vi "Teleop.vi"(10 "Match Info":T1={"Autonomous Elapsed Seconds"=0.0, "TeleOp Elapsed Seconds"=0.0, "Disabled Elapsed Seconds"=0.0, "Visited Autonomous"=FALSE, "Visited TeleOp"=FALSE, "Visited Disabled"=FALSE, "Autonomous Settings"={"Autonomous Style"=enum."Independent", "VI Refnum"=refnum}}, 11 "Call Context":T2) -> ()   [LabVIEW 2020]
doc: "This VI is called for each TeleOp packet received from the DS where the robot is not disabled. It is often used to read from the joysticks and update I/O or to update setpoints for timed control loops. It should complete and return within 20 milliseconds or it may miss DS packets."
uses:
  <vilib>/Rock Robotics/WPI/DriverStation/WPI_DriverStationDerivedRobotMode.ctl
  <vilib>/Rock Robotics/WPI/DriverStation/WPI_DriverStationMatch Info.ctl
  <vilib>/Rock Robotics/WPI/Joystick/XBox Buttons Indexer.ctl
  <vilib>/Rock Robotics/WPI/Joystick/XBox Axes Indexer.ctl
  <vilib>/Rock Robotics/Network Tables/NT Read Boolean.vi
  <vilib>/Rock Robotics/Network Tables/NT Read Number.vi
  Auxilary/AuxGlobals.vi
  Climb/ClimbGlobals.vi
  <vilib>/Rock Robotics/Network Tables/NT Write String.vi
  Human/HumanGlobal.vi
  <vilib>/Rock Robotics/Network Tables/NT Write Boolean.vi
  <vilib>/Rock Robotics/WPI/Joystick/WPI_JoystickArcadeMapping.vi
  <vilib>/Rock Robotics/WPI/ThirdParty/JAS_Junk/TrajLib/Trajectory_Library.lvlib
panel:
  out "Sample Slider 0":dbl(slide) scale=0.0..5.0
  out "Sample Boolean 1":bool
  out "Sample Boolean 0":bool
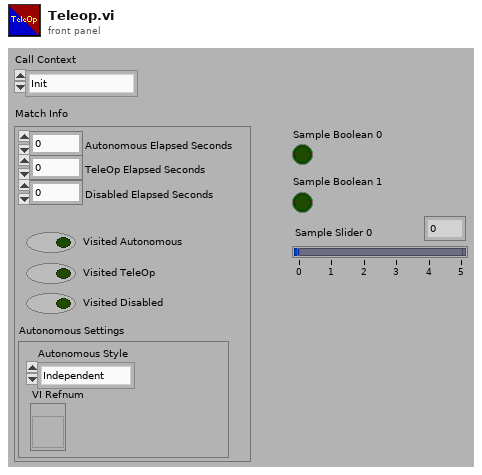
[diagram p1: front panel]
types:
  T1 = typedef "WPI_DriverStationMatch Info.ctl" = cluster{"Autonomous Elapsed Seconds":dbl, "TeleOp Elapsed Seconds":dbl, "Disabled Elapsed Seconds":dbl, "Visited Autonomous":bool, "Visited TeleOp":bool, "Visited Disabled":bool, "Autonomous Settings":cluster{"Autonomous Style":enum16{"Iterative", "Independent"}, "VI Refnum":refnum<vi>}}
  T2 = typedef "WPI_DriverStationDerivedRobotMode.ctl" = enum16{"Init", "Execute", "Stop"}
  T3 = typedef "XBox Buttons Indexer.ctl" = enum16{"A", "B", "X", "Y", "Left Bumper", "Right Bumper", "Back", "Start", "Left Joystick", "Right Joystick"}
  T4 = typedef "XBox Axes Indexer.ctl" = enum16{"Left X", "Left Y", "Left Trigger", "Right Trigger", "Right X", "Right Y"}
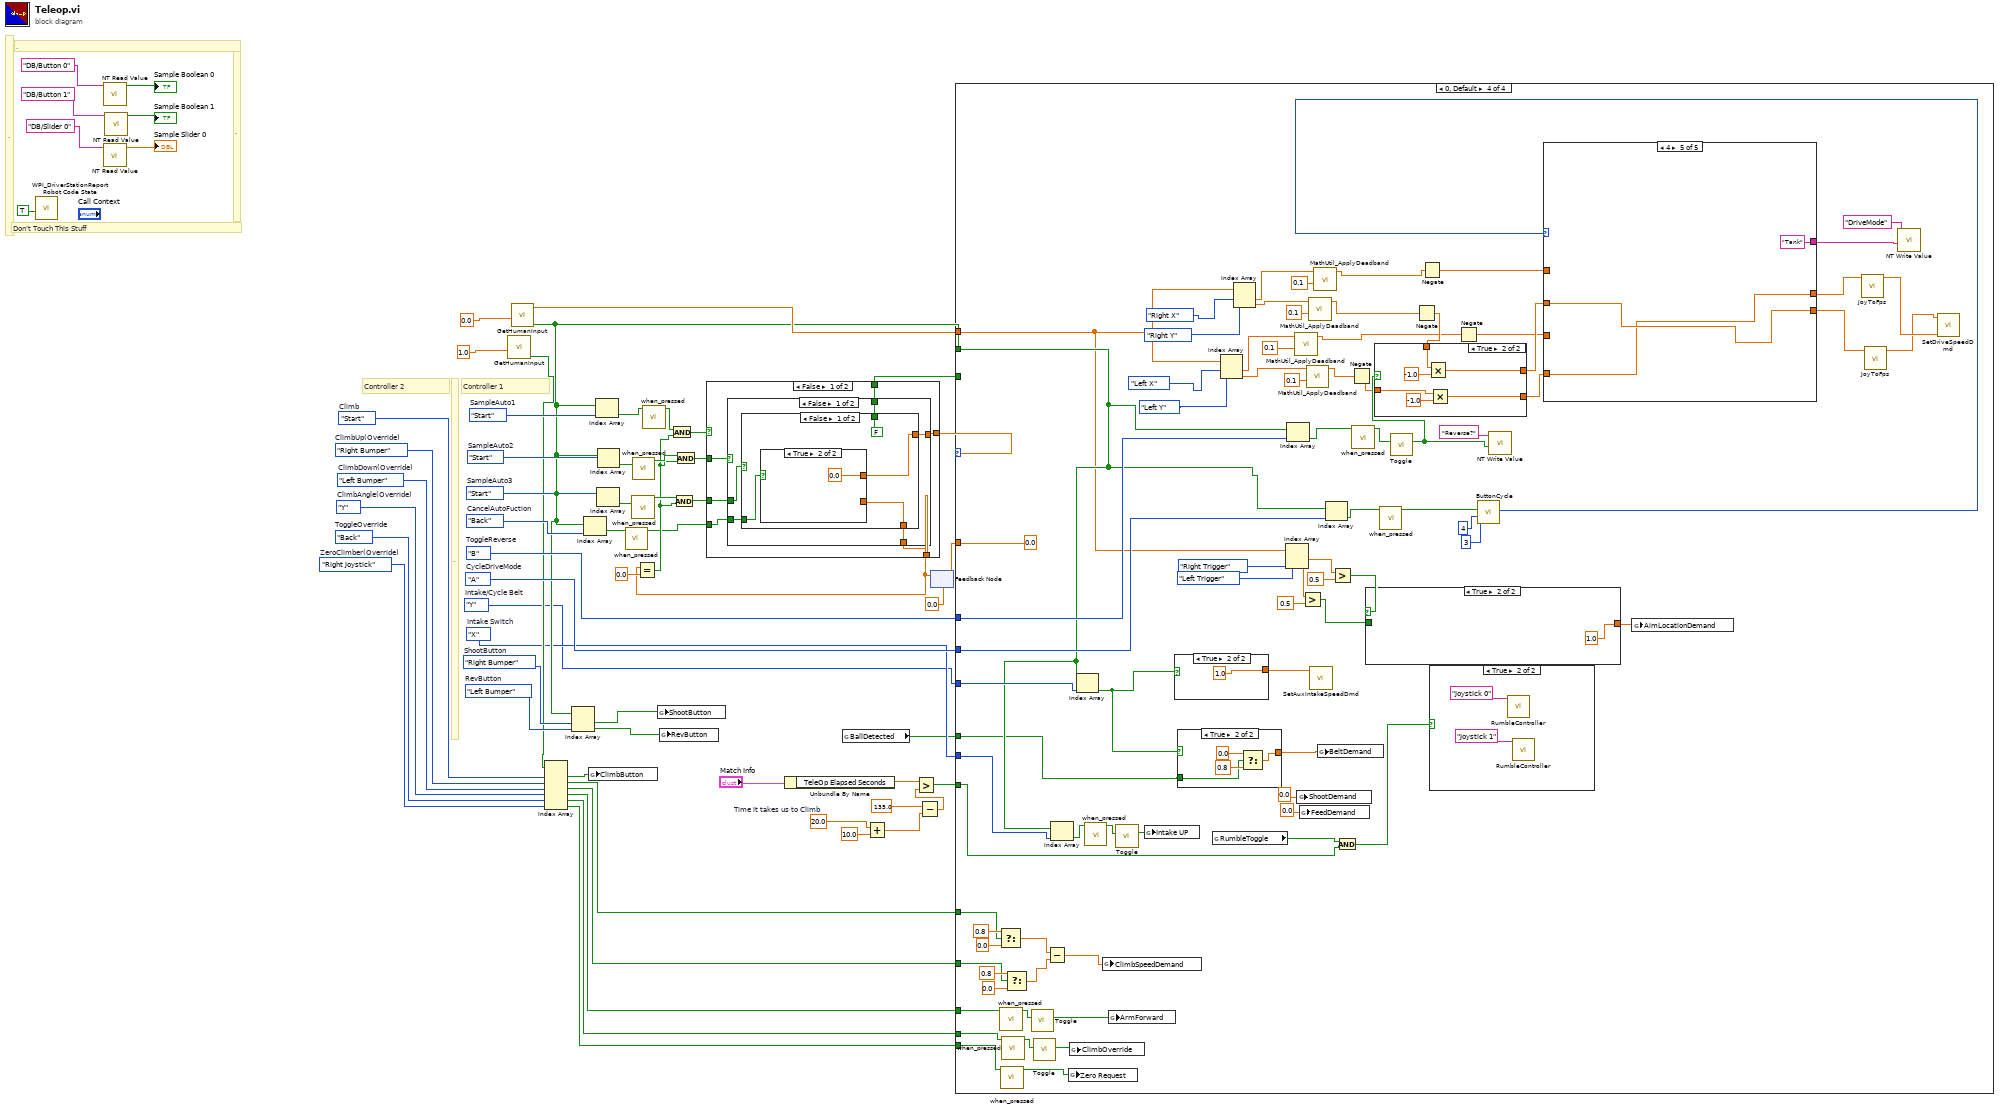
[diagram p0: block diagram]
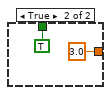
[diagram p3: hidden frame]
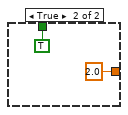
[diagram p4: hidden frame]
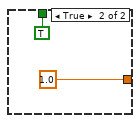
[diagram p5: hidden frame]
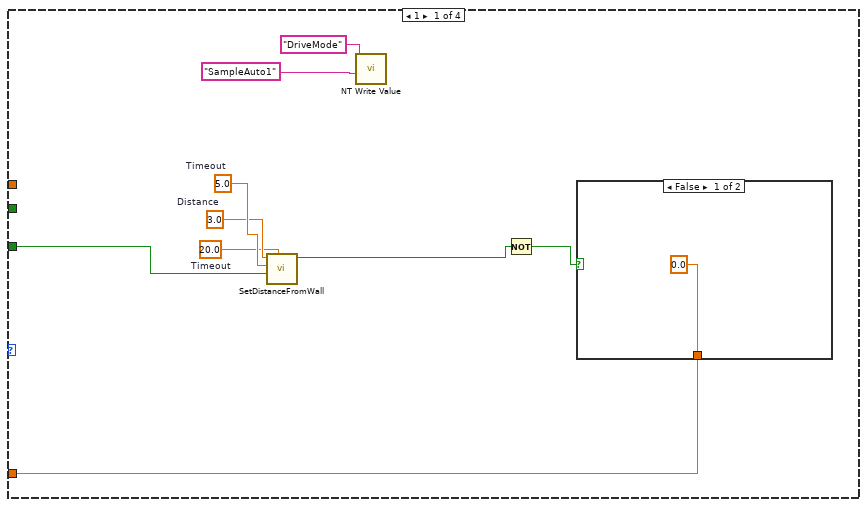
[diagram p6: hidden frame]
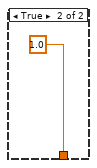
[diagram p7: hidden frame]
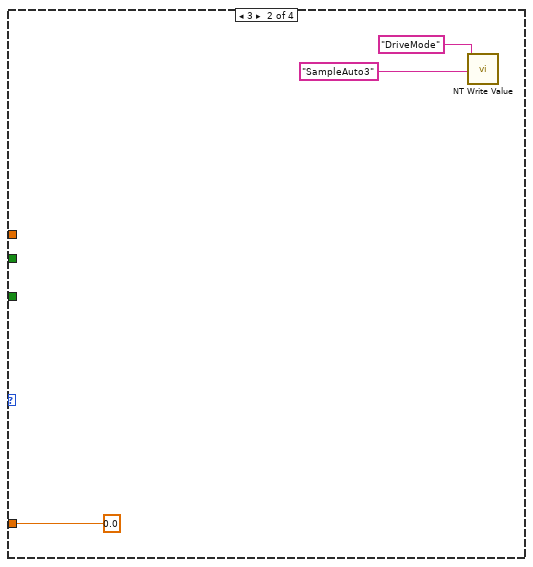
[diagram p8: hidden frame]
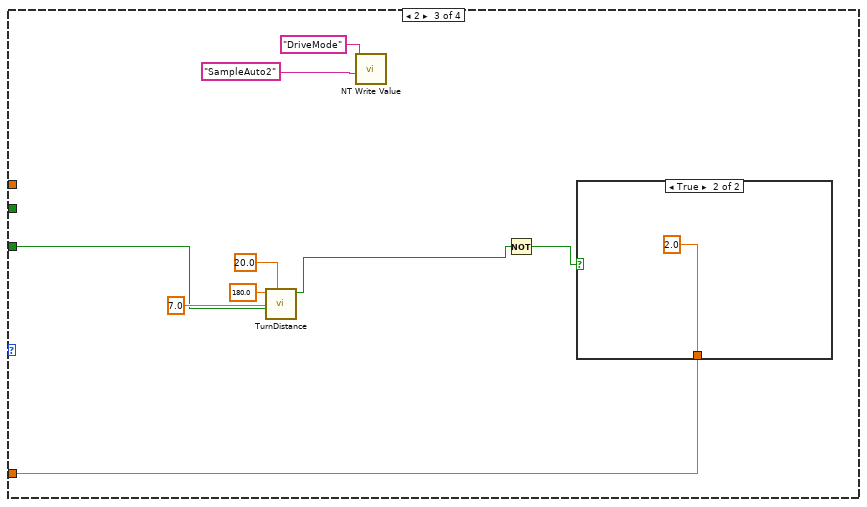
[diagram p9: hidden frame]
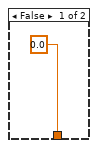
[diagram p10: hidden frame]
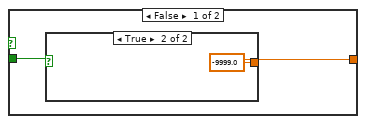
[diagram p11: hidden frame]
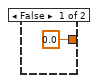
[diagram p12: hidden frame]
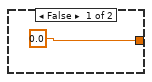
[diagram p13: hidden frame]
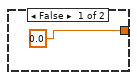
[diagram p14: hidden frame]
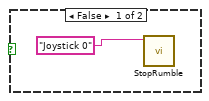
[diagram p15: hidden frame]
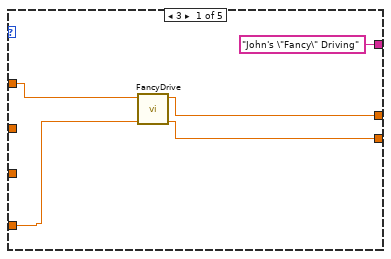
[diagram p17: hidden frame]
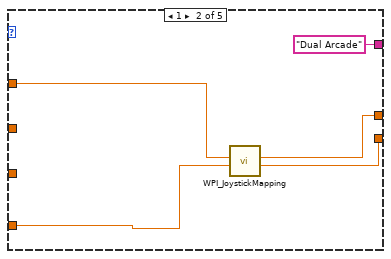
[diagram p18: hidden frame]
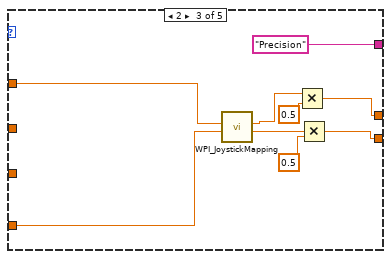
[diagram p19: hidden frame]
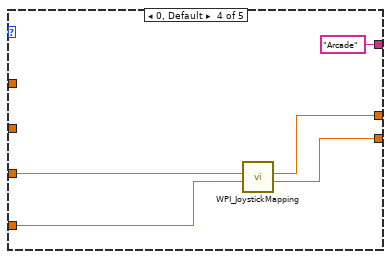
[diagram p20: hidden frame]
diagram:
  w2 = XBox_Buttons_Indexer."Right Joystick"  # ZeroClimber(Override)
  w4 = XBox_Buttons_Indexer."Back"  # ToggleOverride
  w5 = XBox_Buttons_Indexer."Y"  # ClimbAngle(Override)
  w11 = XBox_Buttons_Indexer."Left Bumper"  # ClimbDown(Override)
  w12 = XBox_Buttons_Indexer."Right Bumper"  # ClimbUp(Override)
  w13 = XBox_Buttons_Indexer."Start"  # Climb
  w15 = XBox_Buttons_Indexer."X"  # Intake Switch
  w8 = XBox_Buttons_Indexer."Y"  # Intake/Cycle Belt
  w27 = 20.0  # Time it takes us to Climb
  w18 = XBox_Buttons_Indexer."Left Bumper"  # RevButton
  w19 = XBox_Buttons_Indexer."Right Bumper"  # ShootButton
  w30 = XBox_Buttons_Indexer."A"  # CycleDriveMode
  w31 = XBox_Buttons_Indexer."B"  # ToggleReverse
  w32 = XBox_Buttons_Indexer."Back"  # CancelAutoFuction
  w33 = XBox_Buttons_Indexer."Start"  # SampleAuto3
  w34 = XBox_Buttons_Indexer."Start"  # SampleAuto2
  w35 = XBox_Buttons_Indexer."Start"  # SampleAuto1
  # "."
  # "Controller 2"
  # "Controller 1"
  # "."
  # "."
  # "."
  # "Don't Touch This Stuff"
  n1 = call <vilib>:"WPI_DriverStationReport Robot Code State.vi"("TeleOp"=TRUE ("Autonomous")) -> ()  [unwired: 10 in, 1 out]
  n2 = call-poly <vilib>:"NT Read Value.vi"("Name"="DB/Button 0" ("refnum name")) -> ("Boolean"=→"Sample Boolean 0":bool)  [unwired: 9 in, 1 out]
  n3 = call-poly <vilib>:"NT Read Value.vi"("Name"="DB/Slider 0" ("refnum name")) -> ("Numeric"=→"Sample Slider 0":dbl)  [unwired: 9 in, 1 out]
  n4 = call-poly <vilib>:"NT Read Value.vi"("Name"="DB/Button 1" ("refnum name")) -> ("Boolean"=→"Sample Boolean 1":bool)  [unwired: 9 in, 1 out]
  n5 = call "GetHumanInput.vi"("Controller"=1.0) -> ("Buttons"=w16:bool[])  [unwired: 9 in, 1 out]
  n6 = call "GetHumanInput.vi"("Controller"=0.0) -> ("Buttons"=w20:bool[], "Axes"=w55:dbl[])  [unwired: 9 in]
  n7 = Index Array(array=w16, index #1=w13, index #2=w12, index #3=w11, index #4=w5, index #5=w4, index #6=w2) -> (element #1=w14:bool, element #2=w10:bool, element #3=w9:bool, element #4=w6:bool, element #5=w3:bool, element #6=w1:bool)
  n8 = Index Array(array=w20, index #1=w19, index #2=w18) -> (element #1=w21:bool, element #2=w22:bool)
  n9 = Index Array(array=w20, index=w32) -> (element=w37:bool)
  n10 = global write "ClimbGlobals.vi" "ClimbButton"(w14) -> ()
  n11 = Index Array(array=w20, index=w35) -> (element=w53:bool)
  n12 = Index Array(array=w20, index=w33) -> (element=w48:bool)
  n13 = Index Array(array=w20, index=w34) -> (element=w49:bool)
  n14 = call "when_pressed.vi"("Input"=w37) -> ("Output"=w36:bool)  [unwired: 10 in]
  n15 = call "when_pressed.vi"("Input"=w48) -> ("Output"=w41:bool)  [unwired: 10 in]
  n16 = call "when_pressed.vi"("Input"=w49) -> ("Output"=w40:bool)  [unwired: 10 in]
  n17 = call "when_pressed.vi"("Input"=w53) -> ("Output"=w44:bool)  [unwired: 10 in]
  n18 = global write "AuxGlobals.vi" "ShootButton"(w21) -> ()
  n19 = global write "AuxGlobals.vi" "RevButton"(w22) -> ()
  n20 = Unbundle By Name("Match Info") -> ("TeleOp Elapsed Seconds"=w29:dbl)
  n21 = global read "AuxGlobals.vi" "BallDetected"() -> (w7:bool)
  n22 = Add(x=w27, y=10.0) -> (x+y=w25:dbl)
  n23 = Subtract(x=135.0 ("y"), y=w25) -> (x-y=w24:dbl)
  n24 = Greater?(x=w29, y=w24) -> (0:w23:bool)
  n25 = feedback #1(0.0) -> (w46:dbl)
  n26 = Equal?(x=w46, y=0.0) -> (x = y?=w39:bool)
  n27 = And(x=w44, y=w39) -> (x .and. y?=w45:bool)
  n28 = And(x=w41, y=w39) -> (x .and. y?=w42:bool)
  n29 = And(x=w40, y=w39) -> (x .and. y?=w43:bool)
  n30 = case shown="False" w45 {
    tunnel: [w66 1.0] -> w52
    tunnel: w46 -> [w67 _]
    tunnel: w43 -> [w69 _]
    tunnel: w42 -> [w68 _]
    tunnel: [w65 TRUE] -> w38
    tunnel: w36 -> [w64 _]
    frame False {
      n31 = case shown="False" w69 {
        tunnel: w68 -> [w74 _]
        tunnel: w67 -> [w73 _]
        tunnel: [w72 2.0] -> w66
        tunnel: [w71 TRUE] -> w65
        tunnel: w64 -> [w70 _]
        frame False {
          n32 = case shown="False" w74 {
            tunnel: w73 -> [w75 _]
            tunnel: [w76 3.0] -> w72
            tunnel: [FALSE TRUE] -> w71
            tunnel: w70 -> [w77 _]
            frame False {
              n33 = case shown="True" w77 {
                tunnel: [w79 0.0] -> w76
                tunnel: w75 -> [w79 _]
                frame False {
                }
                frame True {
                }
              }
            }
            frame True {
            }
          }
        }
        frame True {
        }
      }
    }
    frame True {
    }
  }
  n34 = case shown="0, Default" w52 {
    tunnel: w55 -> [_ _ _ w139]
    tunnel: w20 -> [_ _ _ w160]
    tunnel: [w88 0.0 w106 0.0] -> w51
    tunnel: w38 -> [w87 _ w101 _]
    tunnel: w31 -> [_ _ _ w168]
    tunnel: w30 -> [_ _ _ w167]
    tunnel: w23 -> [_ _ _ w163]
    tunnel: w8 -> [_ _ _ w165]
    tunnel: w15 -> [_ _ _ w159]
    tunnel: w10 -> [_ _ _ w127]
    tunnel: w9 -> [_ _ _ w126]
    tunnel: w7 -> [_ _ _ w122]
    tunnel: w6 -> [_ _ _ w117]
    tunnel: w3 -> [_ _ _ w115]
    tunnel: w1 -> [_ _ _ w113]
    frame 1 {
      w91 = 20.0  # Timeout
      w92 = 3.0  # Distance
      w93 = 5.0  # Timeout
      n35 = call "SetDistanceFromWall.vi"("Timeout"=w91, "Initation?"=w87, "MaxSpeed"=w93, "Distance"=w92) -> ("Finished"=w90:bool)  [unwired: 5 in, 2 out]
      n36 = call-poly <vilib>:"NT Write Value.vi"("String"="SampleAuto1", "Name"="DriveMode") -> ()  [unwired: 9 in, 1 out]
      n37 = Not(x=w90) -> (.not. x?=w89:bool)
      n38 = case shown="False" w89 {
        tunnel: [0.0 1.0] -> w88
        frame False {
        }
        frame True {
        }
      }
    }
    frame 3 {
      n39 = call-poly <vilib>:"NT Write Value.vi"("String"="SampleAuto3", "Name"="DriveMode") -> ()  [unwired: 9 in, 1 out]
    }
    frame 2 {
      n40 = call "TurnDistance.vi"("Timeout"=20.0, "Initation?"=w101, "MaxSpeed"=7.0, "Degrees"=180.0) -> ("Finished"=w105:bool)  [unwired: 5 in, 2 out]
      n41 = call-poly <vilib>:"NT Write Value.vi"("String"="SampleAuto2", "Name"="DriveMode") -> ()  [unwired: 9 in, 1 out]
      n42 = Not(x=w105) -> (.not. x?=w107:bool)
      n43 = case shown="True" w107 {
        tunnel: [0.0 2.0] -> w106
        frame False {
        }
        frame True {
        }
      }
    }
    frame 0, Default {
      n44 = Select(t=0.8, s=w127, f=0.0) -> (s? t:f=w124:dbl)
      n45 = call "when_pressed.vi"("Input"=w117) -> ("Output"=w119:bool)  [unwired: 10 in]
      n46 = call "when_pressed.vi"("Input"=w113) -> ("Output"=w112:bool)  [unwired: 10 in]
      n47 = call "when_pressed.vi"("Input"=w115) -> ("Output"=w116:bool)  [unwired: 10 in]
      n48 = Select(t=0.8, s=w126, f=0.0) -> (s? t:f=w125:dbl)
      n49 = call "Toggle.vi"("FlashInput"=w119) -> ("On/Off"=w118:bool)  [unwired: 10 in]
      n50 = call "Toggle.vi"("FlashInput"=w116) -> ("On/Off"=w114:bool)  [unwired: 10 in]
      n51 = Subtract(x=w124, y=w125) -> (x-y=w123:dbl)
      n52 = Index Array(array=w160, index=w159) -> (element=w157:bool)
      n53 = global write "ClimbGlobals.vi" "Zero Request"(w112) -> ()
      n54 = global write "ClimbGlobals.vi" "ClimbOverride"(w114) -> ()
      n55 = Index Array(array=w160, index=w165) -> (element=w121:bool)
      n56 = call "when_pressed.vi"("Input"=w157) -> ("Output"=w158:bool)  [unwired: 10 in]
      n57 = global write "ClimbGlobals.vi" "ClimbSpeedDemand"(w123) -> ()
      n58 = global write "ClimbGlobals.vi" "ArmForward"(w118) -> ()
      n59 = call "Toggle.vi"("FlashInput"=w158) -> ("On/Off"=w161:bool)  [unwired: 10 in]
      n60 = global write "AuxGlobals.vi" "Intake UP"(w161) -> ()
      n61 = case shown="True" w121 {
        tunnel: [0.0 ("Shooter Demand") 1.0 ("Shooter Demand")] -> w166
        frame False {
        }
        frame True {
        }
      }
      n62 = case shown="True" w121 {
        tunnel: [0.0 ("Shooter Demand") w202] -> w156
        tunnel: w122 -> [_ w200]
        frame False {
        }
        frame True {
          n63 = Select(t=0.0 ("Shooter Demand"), s=w200, f=0.8) -> (s? t:f=w202:dbl)
        }
      }
      n64 = global read "HumanGlobal.vi" "RumbleToggle"() -> (w164:bool)
      n65 = Index Array(array=w139, index #1=XBox_Axes_Indexer."Left X" ("XBox Axes"), index #2=XBox_Axes_Indexer."Left Y" ("XBox Axes")) -> (element #1=w145:dbl, element #2=w142:dbl)
      n66 = Index Array(array=w139, index #1=XBox_Axes_Indexer."Right X" ("XBox Axes"), index #2=XBox_Axes_Indexer."Right Y" ("XBox Axes")) -> (element #1=w151:dbl, element #2=w148:dbl)
      n67 = Index Array(array=w139, index #1=XBox_Axes_Indexer."Right Trigger" ("XBox Axes"), index #2=XBox_Axes_Indexer."Left Trigger" ("XBox Axes")) -> (element #1=w138:dbl, element #2=w133:dbl)
      n68 = Index Array(array=w160, index=w168) -> (element=w186:bool)
      n69 = call <vilib>:"MathUtil_ApplyDeadband.vi"("Deadband"=0.1, "Value"=w145) -> ("Result"=w146:dbl)  [unwired: 9 in]
      n70 = global write "AuxGlobals.vi" "ShootDemand"(0.0 ("ShootDemand")) -> ()
      n71 = global write "AuxGlobals.vi" "FeedDemand"(0.0 ("FeedDemand")) -> ()
      n72 = Greater?(x=w133, y=0.5) -> (0:w134:bool)
      n73 = call <vilib>:"MathUtil_ApplyDeadband.vi"("Deadband"=0.1, "Value"=w142) -> ("Result"=w143:dbl)  [unwired: 9 in]
      n74 = call <vilib>:"MathUtil_ApplyDeadband.vi"("Deadband"=0.1, "Value"=w148) -> ("Result"=w149:dbl)  [unwired: 9 in]
      n75 = call "SetAuxIntakeSpeedDmd.vi"("IntakeDemand"=w166) -> ()  [unwired: 11 in]
      n76 = call <vilib>:"MathUtil_ApplyDeadband.vi"("Deadband"=0.1, "Value"=w151) -> ("Result"=w152:dbl)  [unwired: 9 in]
      n77 = global write "AuxGlobals.vi" "BeltDemand"(w156) -> ()
      n78 = Index Array(array=w160, index=w167) -> (element=w192:bool)
      n79 = Greater?(x=w138, y=0.5) -> (0:w136:bool)
      n80 = And(x=w164, y=w163) -> (x .and. y?=w162:bool)
      n81 = Negate(x=w143) -> (-x=w177:dbl)
      n82 = call "when_pressed.vi"("Input"=w186) -> ("Output"=w184:bool)  [unwired: 10 in]
      n83 = case shown="True" w136 {
        tunnel: w134 -> [w194 _]
        tunnel: [w195 1.0] -> w132
        frame False {
          n84 = case shown="True" w194 {
            tunnel: [0.0 -9999.0] -> w195
            frame False {
            }
            frame True {
            }
          }
        }
        frame True {
        }
      }
      n85 = call "when_pressed.vi"("Input"=w192) -> ("Output"=w176:bool)  [unwired: 10 in]
      n86 = call "Toggle.vi"("FlashInput"=w184) -> ("On/Off"=w182:bool)  [unwired: 10 in]
      n87 = Negate(x=w149) -> (-x=w179:dbl)
      n88 = case shown="True" w182 {
        tunnel: w179 -> [w210 w215]
        tunnel: w177 -> [w209 w213]
        tunnel: [w209 w212] -> w183
        tunnel: [w210 w211] -> w181
        frame False {
        }
        frame True {
          n89 = Multiply(x=w215, y=-1.0) -> (x*y=w211:dbl)
          n90 = Multiply(x=w213, y=-1.0) -> (x*y=w212:dbl)
        }
      }
      n91 = Negate(x=w152) -> (-x=w180:dbl)
      n92 = case shown="True" w162 {
        frame False {
          n93 = call "StopRumble.vi"("Controller Name"="Joystick 0") -> ()  [unwired: 11 in]
        }
        frame True {
          n94 = call "RumbleController.vi"("Controller Name"="Joystick 0") -> ()  [unwired: 11 in]
          n95 = call "RumbleController.vi"("Controller Name"="Joystick 1") -> ()  [unwired: 11 in]
        }
      }
      n96 = Negate(x=w146) -> (-x=w178:dbl)
      n97 = call "ButtonCycle.vi"("Start At"=3, "MaxNum"=4, "FlashInput"=w176) -> ("CycleNumber"=w175:i32)  [unwired: 8 in]
      n98 = call-poly <vilib>:"NT Write Value.vi"("Boolean"=w182, "Name"="Reverse?") -> ()  [unwired: 9 in, 1 out]
      n99 = case shown="4" w175 {
        tunnel: w178 -> [_ _ _ w240 _]
        tunnel: w183 -> [w219 w224 w234 w239 w241]
        tunnel: [w217 w225 w228 w238 w241] -> w191
        tunnel: [w218 w226 w227 w237 w242] -> w190
        tunnel: w180 -> [w220 w223 w235 _ _]
        tunnel: ["John's \"Fancy\" Driving" "Dual Arcade" "Precision" "Arcade" "Tank"] -> w187
        tunnel: w181 -> [_ _ _ _ w242]
        frame 3 {
          n100 = call "FancyDrive.vi"("Y axis value"=w219, "X axis value"=w220) -> ("Right Motor Value"=w218:dbl, "Left Motor Value"=w217:dbl)  [unwired: 8 in]
        }
        frame 1 {
          n101 = call-poly <vilib>:"WPI_JoystickMapping.vi"("Y axis value"=w224, "X axis value"=w223) -> ("Right Motor Value"=w226:dbl, "Left Motor Value"=w225:dbl)  [unwired: 8 in]
        }
        frame 2 {
          n102 = call-poly <vilib>:"WPI_JoystickMapping.vi"("Y axis value"=w234, "X axis value"=w235) -> ("Right Motor Value"=w232:dbl, "Left Motor Value"=w231:dbl)  [unwired: 8 in]
          n103 = Multiply(x=w231, y=0.5) -> (x*y=w228:dbl)
          n104 = Multiply(x=w232, y=0.5) -> (x*y=w227:dbl)
        }
        frame 0, Default {
          n105 = call-poly <vilib>:"WPI_JoystickMapping.vi"("Y axis value"=w239, "X axis value"=w240) -> ("Right Motor Value"=w237:dbl, "Left Motor Value"=w238:dbl)  [unwired: 8 in]
        }
        frame 4 {
        }
      }
      n106 = global write "AuxGlobals.vi" "AimLocationDemand"(w132) -> ()
      n107 = call "JoyToFps.vi"("JoystickInput"=w191) -> ("Fps"=w189:dbl)  [unwired: 10 in]
      n108 = call "JoyToFps.vi"("JoystickInput"=w190) -> ("Fps"=w188:dbl)  [unwired: 10 in]
      n109 = call-poly <vilib>:"NT Write Value.vi"("String"=w187, "Name"="DriveMode") -> ()  [unwired: 9 in, 1 out]
      n110 = call "SetDriveSpeedDmd.vi"("LeftSpeedInput"=w189, "RightSpeedInput"=w188) -> ()  [unwired: 10 in]
    }
  }
  n111 = feedback-in #1(w51) -> ()
